vi "QueryServer_StartServer.vi"(5 "Server Key File (.key)":path, 7 "Server Certificate File (.crt)":path, 8 "error in (no error)":errorcluster, 10 "gRPCid":T1, 11 "Server Address":string) -> (0 "error out":errorcluster)   [LabVIEW 2019, in "labview-grpc-query-server.lvlib"]
uses:
  labview-grpc-query-server.lvlib
  QueryServer_gRPCid.ctl
  <vilib>/Utility/error.llb/Error Cluster From Error Code.vi
  <vilib>/ErrorRing/Error Ring.xnode
  build/Debug/labview_measurement_server.dll
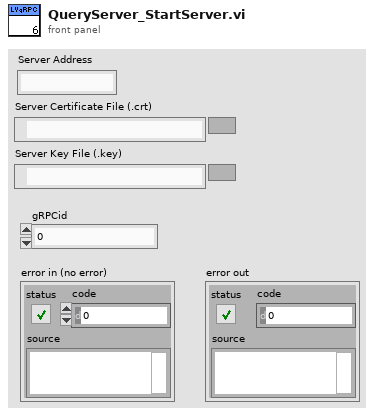
[diagram p1: front panel]
types:
  T1 = typedef "labview-grpc-query-server.lvlib/QueryServer_gRPCid.ctl" = u64
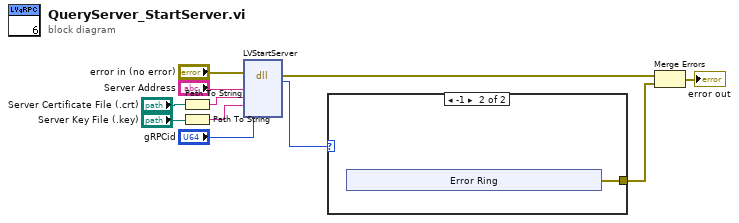
[diagram p0: block diagram]
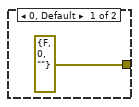
[diagram p2: hidden frame]
diagram:
  n1 = Path To String(path="Server Certificate File (.crt)") -> (string=w8:string)
  n2 = Path To String(path="Server Key File (.key)") -> (string=w7:string)
  n3 = dll-call lib="C:/dev/labview-grpc-measurement-server/build/Debug/labview_measurement_server.dll" fn="LVStartServer"(error in="error in (no error)", "serveraddress"="Server Address", "serverCertificateFile"=w8, "serverKeyFile"=w7, "serverid"="gRPCid") -> (error out=w1:errorcluster, "return type"=w4:i32)  [unwired: 6 in, 1 out]
  n4 = case shown="-1" w4 {
    tunnel: [errorcluster {"status"=FALSE, "code"=0, "source"=""} ("error constant") w13] -> w2
    frame 0, Default {
    }
    frame -1 {
      n5 = xnode "Error Ring"() -> ("error out"=w13:errorcluster)
    }
  }
  n6 = Merge Errors(w1, w2) -> (→"error out":errorcluster)
